vi "GDSString_XML_GetTagBlock.vi"(1 "TextIn":string, 2 "TagName":string, 3 "AttributeName":string, 4 "offset (0)":i32, 5 "error in (no error)":errorcluster) -> (12 "AttributeString":string, 14 "TagName":string, 15 "TextWithinTag":string, 16 "AttributeValue":string, 17 "TextAfterTag":string, 18 "OffsetPastThisTag":i32, 19 "error out":errorcluster)   [LabVIEW 2020]
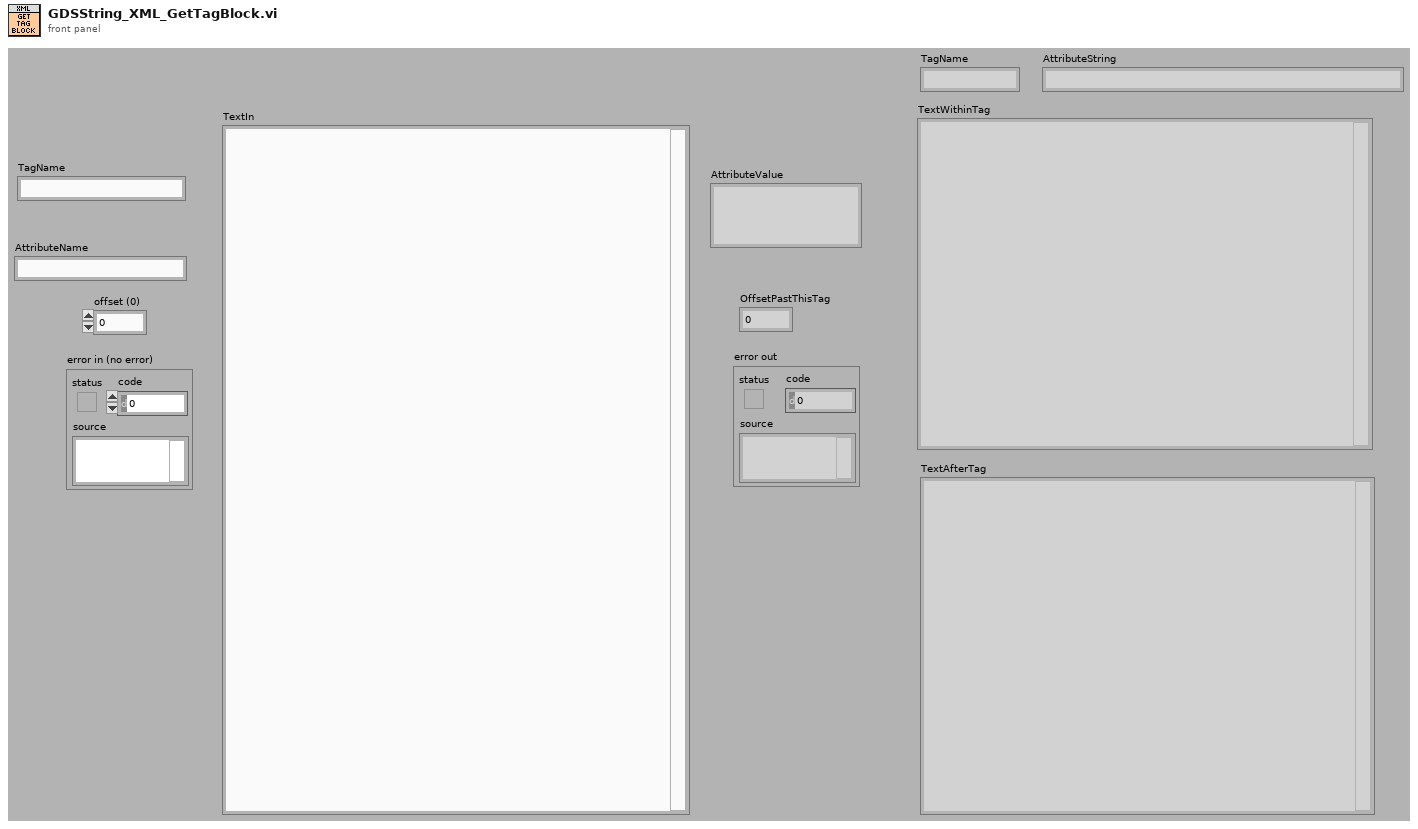
[diagram p1: front panel]
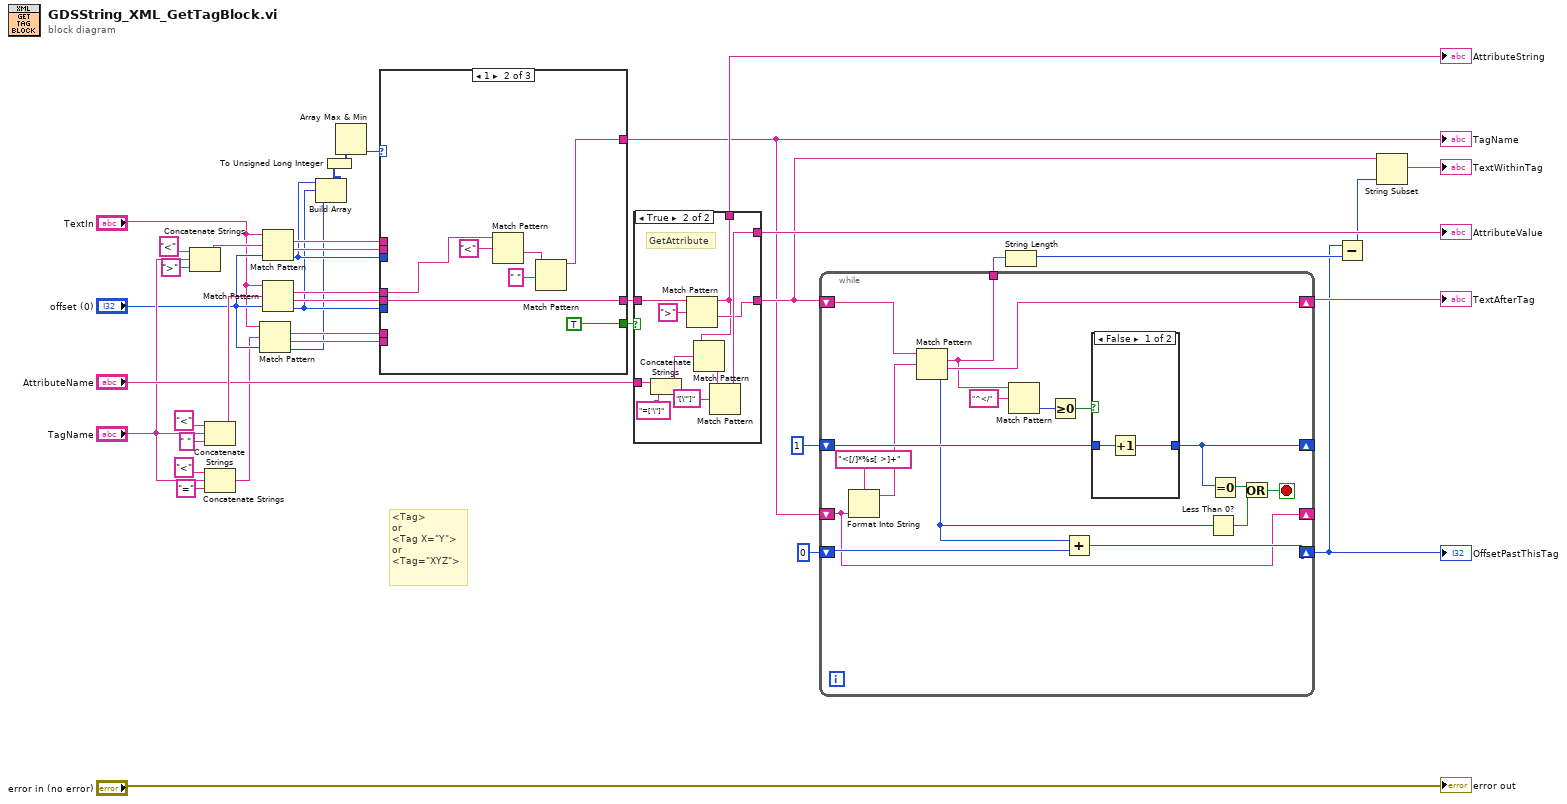
[diagram p0: block diagram]
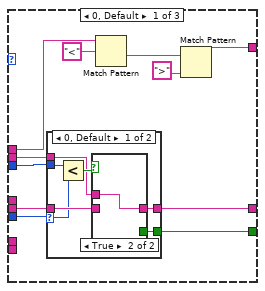
[diagram p2: hidden frame]
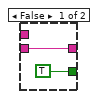
[diagram p3: hidden frame]
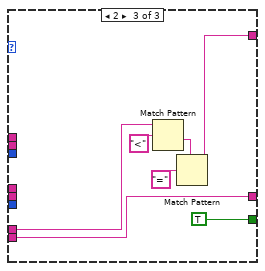
[diagram p5: hidden frame]
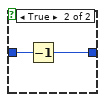
[diagram p6: hidden frame]
diagram:
  # "<Tag>\nor\n<Tag X=\"Y\">\nor\n<Tag=\"XYZ\">"
  n1 = Concatenate Strings("<" ("regular expression"), "TagName", ">" ("string")) -> (w34:string)
  n2 = Concatenate Strings("<" ("regular expression"), "TagName", " " ("string")) -> (w40:string)
  n3 = Concatenate Strings("<" ("regular expression"), "TagName", "=" ("string")) -> (w11:string)
  n4 = Match Pattern(string="TextIn", regular expression=w11, offset (0)="offset (0)") -> (match substring=w10:string, after substring=w9:string, offset past match=w6:i32)  [unwired: 1 out]
  n5 = Match Pattern(string="TextIn", regular expression=w34, offset (0)="offset (0)") -> (match substring=w15:string, after substring=w32:string, offset past match=w8:i32)  [unwired: 1 out]
  n6 = Match Pattern(string="TextIn", regular expression=w40, offset (0)="offset (0)") -> (match substring=w14:string, after substring=w33:string, offset past match=w7:i32)  [unwired: 1 out]
  n7 = Build Array(w8, w7, w6) -> (w5:i32[])
  n8 = To Unsigned Long Integer(number=w5) -> (unsigned 32bit integer=w3:u32[])
  n9 = Array Max & Min(array=w3) -> (min index (indices)=w4:i32)  [unwired: 3 out]
  n10 = case shown="1" w4 {
    tunnel: w33 -> [w51 w68 _]
    tunnel: w32 -> [w50 _ _]
    tunnel: [w49 TRUE TRUE] -> w31
    tunnel: [w48 w68 w73] -> w30
    tunnel: [w47 w67 w75] -> w1
    tunnel: w15 -> [w46 _ _]
    tunnel: w14 -> [_ w66 _]
    tunnel: w10 -> [_ _ w74]
    tunnel: w9 -> [_ _ w73]
    tunnel: w8 -> [w45 _ _]
    tunnel: w7 -> [w44 _ _]
    frame 0, Default {
      n11 = case shown="0, Default" w44 {
        selector: w44 -> [w53 _]
        tunnel: [w57 w62] -> w48
        tunnel: w50 -> [w56 w62]
        tunnel: w45 -> [w55 _]
        tunnel: w51 -> [w54 _]
        tunnel: [w52 _] -> w49
        frame 0, Default {
          n12 = Less?(x=w55, y=w53) -> (x < y?=w58:bool)
          n13 = case shown="True" w58 {
            tunnel: [w60 w61] -> w57
            tunnel: w56 -> [_ w61]
            tunnel: w54 -> [w60 _]
            tunnel: [TRUE _] -> w52
            frame False {
            }
            frame True {
            }
          }
        }
        frame -1 {
        }
      }
      n14 = Match Pattern(string=w46, regular expression="<") -> (after substring=w42:string)  [unwired: 4 out]
      n15 = Match Pattern(string=w42, regular expression=">") -> (before substring=w47:string)  [unwired: 4 out]
    }
    frame 1 {
      n16 = Match Pattern(string=w66, regular expression="<") -> (after substring=w64:string)  [unwired: 4 out]
      n17 = Match Pattern(string=w64, regular expression=" ") -> (before substring=w67:string)  [unwired: 4 out]
    }
    frame 2 {
      n18 = Match Pattern(string=w74, regular expression="<") -> (after substring=w71:string)  [unwired: 4 out]
      n19 = Match Pattern(string=w71, regular expression="=") -> (before substring=w75:string)  [unwired: 4 out]
    }
  }
  "TagName" <- w1
  n20 = case shown="True" w31 {
    tunnel: w30 -> [w77 w86]
    tunnel: "AttributeName" -> [_ w84]
    tunnel: [_ w80] -> w28
    tunnel: [w77 w79] -> w24
    tunnel: [_ w78] -> w2
    frame False {
    }
    frame True {
      # "GetAttribute"
      n21 = Concatenate Strings(w84, "=['\"]" ("regular expression")) -> (w83:string)
      n22 = Match Pattern(string=w86, regular expression=">") -> (before substring=w78:string, after substring=w79:string)  [unwired: 3 out]
      n23 = Match Pattern(string=w78, regular expression=w83) -> (after substring=w82:string)  [unwired: 4 out]
      n24 = Match Pattern(string=w82, regular expression="[\"']") -> (before substring=w80:string)  [unwired: 4 out]
    }
  }
  "AttributeValue" <- w28
  "AttributeString" <- w2
  n25 = while {
    shift-right: [w103] -> w26
    shift-left: w24 -> [w104]
    shift-right: [w98] -> _
    shift-left: 1 -> [w99]
    shift-right: [w92] -> w17
    shift-left: 0 -> [w93]
    tunnel: [w90] -> w22
    shift-right: [w88] -> _
    shift-left: w1 -> [w88]
    stop <- w96 stop-if-true
    n26 = Format Into String(format string="<[/]*%s[ >]+" ("regular expression"), w88) -> (resulting string=w89:string)  [unwired: 2 in, 1 out]
    n27 = Match Pattern(string=w104, regular expression=w89) -> (match substring=w90:string, after substring=w103:string, offset past match=w94:i32)  [unwired: 2 out]
    n28 = Match Pattern(string=w90, regular expression="^</") -> (offset past match=w101:i32)  [unwired: 4 out]
    n29 = Greater Or Equal To 0?(x=w101) -> (x >= 0?=w100:bool)
    n30 = Add(x=w94, y=w93) -> (x+y=w92:i32)
    n31 = case shown="False" w100 {
      tunnel: w99 -> [w106 w108]
      tunnel: [w105 w107] -> w98
      frame False {
        n32 = Increment(x=w106) -> (x+1=w105:i32)
      }
      frame True {
        n33 = Decrement(x=w108) -> (x-1=w107:i32)
      }
    }
    n34 = Less Than 0?(x=w94) -> (x < 0?=w95:bool)
    n35 = Equal To 0?(x=w98) -> (x = 0?=w97:bool)
    n36 = Or(x=w97, y=w95) -> (x .or. y?=w96:bool)
  }
  "OffsetPastThisTag" <- w17
  "TextAfterTag" <- w26
  n37 = String Length(string=w22) -> (length=w21:i32)
  n38 = Subtract(x=w17, y=w21) -> (x-y=w20:i32)
  n39 = String Subset(string=w24, length (rest)=w20) -> (substring=→"TextWithinTag":string)  [unwired: 1 out]
  "error out" <- "error in (no error)"
